vi "LP Set Slew Speed for 3 axis.vi"(7 "Max Speed":dbl=60000.0, 8 "Yaw Gain":dbl, 9 "Pitch Gain":dbl, 10 "Roll Gain":dbl, 11 "output cluster":T2) -> (0 "error out":errorcluster, 1 "InRange":bool)   [LabVIEW 2015]
uses:
  Controls/LP Motor Thread Data.ctl
  Stream/Controls/LP Axis Closed Loop Data.ctl
  MCode_LV_86/Set Parameter.ctl
  MCode_LV_86/MDrive Mode.ctl
  Stream/LP Globals.vi
panel:
  in  "Wait After CMD":u32=40
  out "Roll Nominal":dbl
  out "IMUdata":dbl[](array[numeric])
  out "Pitch Nominal":dbl
  out "ClosedLoopData":T1
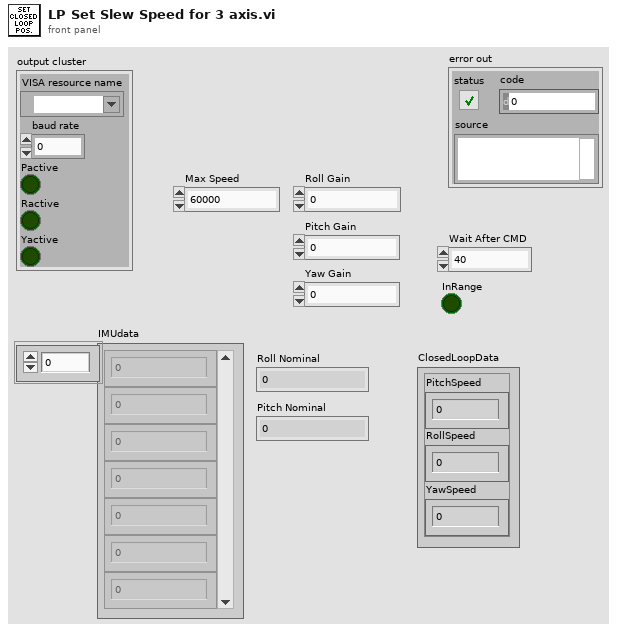
[diagram p1: front panel]
types:
  T1 = typedef "LP Axis Closed Loop Data.ctl" = cluster{"PitchSpeed":dbl, "RollSpeed":dbl, "YawSpeed":dbl}
  T2 = typedef "LP Motor Thread Data.ctl" = cluster{"VISA resource name":refnum<visa-resource-name>, "baud rate":u32, "Pactive":bool, "Ractive":bool, "Yactive":bool}
  T3 = typedef "LP Motor Pos And State.ctl" = cluster{"PosPitch":dbl, "PosRoll":dbl, "PosYaw":dbl, "PitchMov":bool, "RollMov":bool, "YawMov":bool}
  T4 = cluster{"Max Speed":dbl, "Max Speed":dbl, "upper limit":dbl}
  T5 = typedef "MDrive Mode.ctl" = enum16{"Normal Mode", "Party Mode"}
  T6 = typedef "Set Parameter.ctl" = enum16{"Acceleration (A)", "Baud Rate (BD)", "Counter 1 (C1)", "Counter 2 (C2)", "Control C Software Reset (CE)", "Check Sum Enable (CK)", "Clock Mode (CM)", "Clock Mode Ratio (CR)", "Clock Mode Out Step Width (CW)", "Deceleration (D)", "Digital Filtering, Input 1 (D1)", "Digital Filtering, Input 2 (D2)", "Digital Filtering, Input 3 (D3)", "Digital Filtering, Input 4 (D4)", "Digital Filtering, Input 5 (D5)", "Digital Filtering, Input 9 (D9)", "Digital Filtering, Input 10 (D10)", "Digital Filtering, Input 11 (D11)", "Digital Filtering, Input 12 (D12)", "Deadband (DB)", "Decrement Variable (DC)", "Enable/Disable Drive (DE)", "Device Name (DN)", "End Program Execution (E)", "Encoder Function Enable (EE)", "Encoder Lines (EL)", "Echo Mode (EM)", "Error Clear (ER)", "Escape (ES)", "Execute Program at Address (EX)", "Factory Default (FD)", "Hold (H)", "Hold Current (HC)", "Hold Current Encoder Index (HI)", "Home to Home Switch (HM)", "Home to Delay Time (HT)", "Increment Variable (IC)", "Initialize Parameters to NVM (IP)", "Input into Variable (IV)", "Jog Enable (JE)", "Limit Stop Mode (LM)", "Move Absolute (MA)", "Move Relative (MR)", "MicroStepping Select (MS)", "Motor Settling Delay Time (MT)", "Output 1 (O1)", "Output 2 (O2)", "Output 3 (O3)", "Output 4 (O4)", "Output 9 (O9)", "Output 10 (O10)", "Output 11 (O11)", "Output 12 (O12)", "Output High Byte (9-12) (OH)", "Output Low Byte (1-4) (OL)", "Output Total (1-4 and 9-12) (OT)", "Position (P)", "Position Maintenance (PM)", "Party Mode (PY)", "Register 1 (R1)", "Register 2 (R2)", "Register 3 (R3)", "Register 4 (R4)", "Run Current (RC)", "Stall Factor (SF)", "Slew (SL)", "Stall Mode Set (SM)", "Upgrade Firmware (UG)", "Velocity Initial (VI)", "Velocity Maximum (VM)", "Set Input #1 as Home (S1)", "Save (S)", "Save DN+PY (NameS)", "Active Party Mode (0x0A)", "Set Input #1 (S1) as Limit- Active Floating", "Set Input #2 (S2) as Limit+ Active Floating", "Set Input #1 as Home (S1) Active Floating", "Set Input #1 as Home (S2) Active Floating", "Set Input #1 (S1) as Limit+ Active Floating", "Set Input #2 (S2) as Limit- Active Floating", "Hybrid Mode (AS)"}
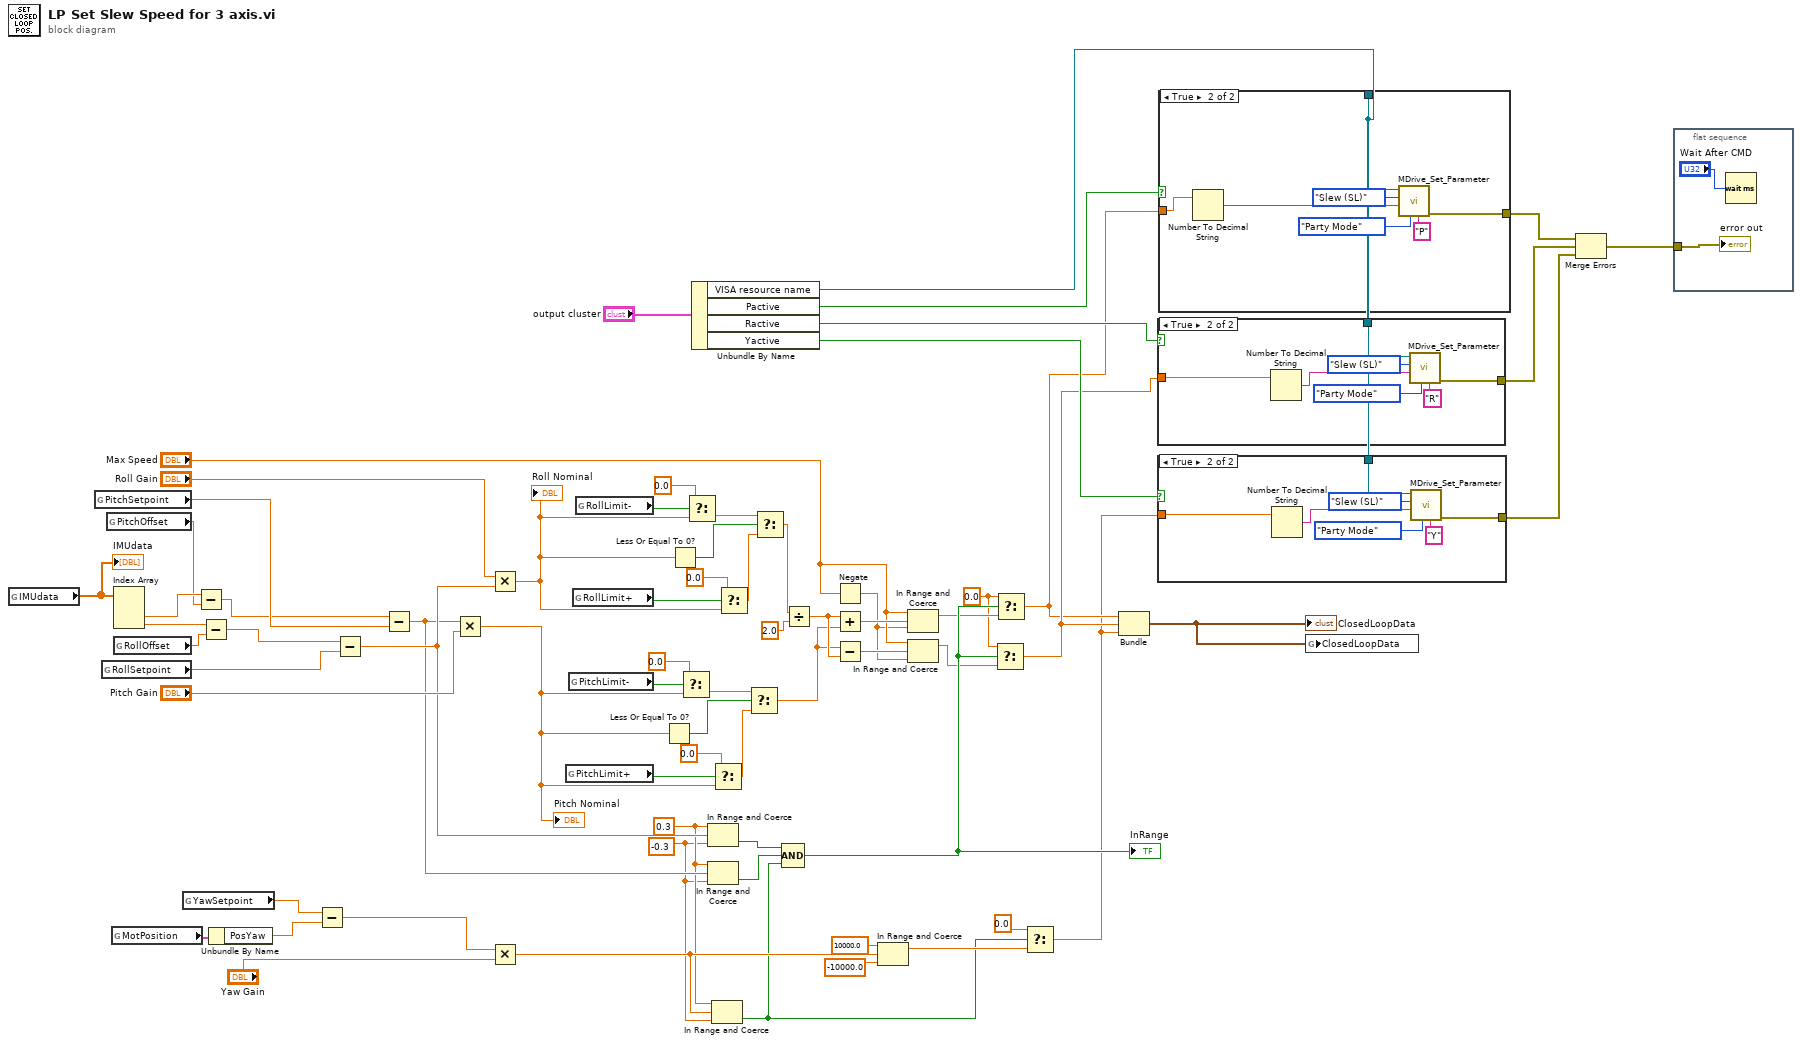
[diagram p0: block diagram]
diagram:
  w15 = 0.0 ("t")
  w5 = -0.3 ("upper limit")
  w6 = 0.3 ("upper limit")
  n1 = global read "LP Globals.vi" "IMUdata"() -> (w64:dbl[])
  "IMUdata" <- w64
  n2 = global read "LP Globals.vi" "PitchSetpoint"() -> (w54:dbl)
  n3 = global read "LP Globals.vi" "RollSetpoint"() -> (w53:dbl)
  n4 = global read "LP Globals.vi" "PitchOffset"() -> (w48:dbl)
  n5 = global read "LP Globals.vi" "MotPosition"() -> (w14:T3)
  n6 = Index Array(array=w64) -> (element #2=w52:dbl, element #3=w50:dbl)  [unwired: 3 in, 1 out]
  n7 = global read "LP Globals.vi" "RollOffset"() -> (w47:dbl)
  n8 = global read "LP Globals.vi" "YawSetpoint"() -> (w13:dbl)
  n9 = Subtract(x=w52, y=w48) -> (x-y=w51:dbl)
  n10 = Subtract(x=w50, y=w47) -> (x-y=w49:dbl)
  n11 = Unbundle By Name(w14) -> ("PosYaw"=w12:dbl)
  n12 = Subtract(x=w13, y=w12) -> (x-y=w11:dbl)
  n13 = Subtract(x=w49, y=w53) -> (x-y=w46:dbl)
  n14 = Subtract(x=w51, y=w54) -> (x-y=w45:dbl)
  n15 = Multiply(x=w45, y="Pitch Gain") -> (x*y=w22:dbl)
  "Pitch Nominal" <- w22
  n16 = Multiply(x="Roll Gain", y=w46) -> (x*y=w31:dbl)
  "Roll Nominal" <- w31
  n17 = Multiply(x=w11, y="Yaw Gain") -> (x*y=w7:dbl)
  n18 = global read "LP Globals.vi" "PitchLimit+"() -> (w28:bool)
  n19 = global read "LP Globals.vi" "PitchLimit-"() -> (w24:bool)
  n20 = global read "LP Globals.vi" "RollLimit+"() -> (w32:bool)
  n21 = global read "LP Globals.vi" "RollLimit-"() -> (w37:bool)
  n22 = Less Or Equal To 0?(x=w22) -> (x <= 0?=w23:bool)
  n23 = Less Or Equal To 0?(x=w31) -> (x <= 0?=w38:bool)
  n24 = Select(t=0.0, s=w24, f=w22) -> (s? t:f=w25:dbl)
  n25 = Select(t=0.0, s=w37, f=w31) -> (s? t:f=w36:dbl)
  n26 = Unbundle By Name("output cluster") -> ("VISA resource name"=w69:refnum<visa-resource-name>, "Pactive"=w66:bool, "Ractive"=w67:bool, "Yactive"=w68:bool)
  n27 = In Range and Coerce(upper limit=w6, x=w46, lower limit=w5) -> (In Range?=w44:bool)  [unwired: 1 out]
  n28 = In Range and Coerce(upper limit=w6, x=w45, lower limit=w5) -> (In Range?=w43:bool)  [unwired: 1 out]
  n29 = In Range and Coerce(upper limit=w6, x=w7, lower limit=w5) -> (In Range?=w1:bool)  [unwired: 1 out]
  n30 = Select(t=0.0, s=w28, f=w22) -> (s? t:f=w29:dbl)
  n31 = Select(t=0.0, s=w32, f=w31) -> (s? t:f=w30:dbl)
  n32 = Select(t=w25, s=w23, f=w29) -> (s? t:f=w21:dbl)
  n33 = Select(t=w36, s=w38, f=w30) -> (s? t:f=w35:dbl)
  n34 = Compound Arithmetic op=AND(w44, w43, w1) -> (w20:bool)
  "InRange" <- w20
  n35 = Divide(x=w35, y=2.0) -> (x/y=w61:dbl)
  n36 = Negate(x="Max Speed") -> (-x=w55:dbl)
  n37 = Add(x=w61, y=w21) -> (x+y=w58:dbl)
  n38 = Subtract(x=w21, y=w61) -> (x-y=w57:dbl)
  n39 = In Range and Coerce(upper limit=10000.0, x=w7, lower limit=-10000.0 ("upper limit")) -> (coerced(x)=w3:dbl)  [unwired: 1 out]
  n40 = In Range and Coerce(upper limit="Max Speed", x=w58, lower limit=w55) -> (coerced(x)=w17:dbl)  [unwired: 1 out]
  n41 = In Range and Coerce(upper limit="Max Speed", x=w57, lower limit=w55) -> (coerced(x)=w19:dbl)  [unwired: 1 out]
  n42 = Select(t=w15, s=w20, f=w19) -> (s? t:f=w18:dbl)
  n43 = Select(t=w15, s=w20, f=w17) -> (s? t:f=w16:dbl)
  n44 = Select(t=0.0, s=w1, f=w3) -> (s? t:f=w2:dbl)
  n45 = Bundle("Max Speed"=w16, "Max Speed"=w18, "upper limit"=w2) -> (w60:T4)  [unwired: 1 in]
  "ClosedLoopData" <- w60
  n46 = case shown="True" w67 {
    tunnel: w69 -> [_ w76]
    tunnel: w18 -> [_ w72]
    tunnel: [_ w70] -> w41
    frame False {
    }
    frame True {
      n47 = Number To Decimal String(number=w72) -> (decimal integer string=w71:string)  [unwired: 1 in]
      n48 = call "MDrive_Set_Parameter.vi"("Device Name"="R", "Mdrive Mode"=MDrive_Mode."Party Mode", "Parameter Setpoint"=w71, "Set Parameter"=Set_Parameter."Slew (SL)", "VISA IN"=w76) -> ("error out"=w70:errorcluster)  [unwired: 4 in, 2 out]
    }
  }
  n49 = case shown="True" w68 {
    tunnel: w69 -> [_ w83]
    tunnel: [_ w78] -> w40
    tunnel: w2 -> [_ w77]
    frame False {
    }
    frame True {
      n50 = Number To Decimal String(number=w77) -> (decimal integer string=w79:string)  [unwired: 1 in]
      n51 = call "MDrive_Set_Parameter.vi"("Device Name"="Y", "Mdrive Mode"=MDrive_Mode."Party Mode", "Parameter Setpoint"=w79, "Set Parameter"=Set_Parameter."Slew (SL)", "VISA IN"=w83) -> ("error out"=w78:errorcluster)  [unwired: 4 in, 2 out]
    }
  }
  n52 = case shown="True" w66 {
    tunnel: w69 -> [_ w90]
    tunnel: w16 -> [_ w89]
    tunnel: [_ w87] -> w42
    frame False {
    }
    frame True {
      n53 = Number To Decimal String(number=w89) -> (decimal integer string=w88:string)  [unwired: 1 in]
      n54 = call "MDrive_Set_Parameter.vi"("Device Name"="P", "Mdrive Mode"=MDrive_Mode."Party Mode", "Parameter Setpoint"=w88, "Set Parameter"=Set_Parameter."Slew (SL)", "VISA IN"=w90) -> ("error out"=w87:errorcluster)  [unwired: 4 in, 2 out]
    }
  }
  n55 = global write "LP Globals.vi" "ClosedLoopData"(w60) -> ()
  n56 = Merge Errors(w42, w41, w40) -> (w39:errorcluster)
  n57 = flat-sequence {
    tunnel: w39 -> [w92]
    frame #0 {
      n58 = Wait (ms)(milliseconds to wait="Wait After CMD") -> ()  [unwired: 1 out]
      "error out" <- w92
    }
  }
